vi "PilotPlant.vi"() -> ()   [LabVIEW 2019]
uses:
  Manual or Auto.ctl
  setpoints.ctl
  backwash.ctl
  coag.ctl
  model type.ctl
  data channels.ctl
  file paths.ctl
  state.ctl
  data ave state.ctl
  ini.ctl
  Sensor buffer command.ctl
  data buffer cmd.ctl
  <vilib>/addons/control/pid/pid.llb/PID (DBL).vi
  <vilib>/addons/control/pid/NI_PID_pid.lvlib
panel:
  in  "Tab Control":enum32{"Graphs", "Controls", "About"}(tab)
  in  "data points to display":u16=100 min=1 step=1
  out "coag":cluster{timestamp[], dbl[]}[](graph)
  out "Misc":cluster{timestamp[], dbl[]}[](graph)
  out "Turbidities":cluster{timestamp[], dbl[]}[](graph)
  out "Sludge valve":dbl(graph)
  out "Plant flow valve":dbl(graph)
  in  "data channel":T1
  out "recent data":dbl[](array[numeric])
  out "out of range":bool
  in  "setpoints":T2={"data update interval (s)"=100.0, "sludge flow [L/s]"=0.0, "plant flow [L/s]"=0.05, "Plant Flow PID "={"proportional gain (Kc)"=0.05, "integral time (Ti, min)"=1.0, "derivative time (Td, min)"=0.01}, "Sludge PID "={"proportional gain (Kc)"=0.07, "integral time (Ti, min)"=1.0, "derivative time (Td, min)"=0.01}, "backwash"={"Filtered quality target [NTU]"=0.3, "min filtration time [s]"=600.0, "Ripen time [s]"=600.0}, "Coagulant"={"flocculator volume (L)"=0.0, "clarifier volume (L)"=0.0, "dose updates per response delay"=100, "target clarified turbidity (NTU)"=0.3, "Coagulant mode"=enum."manual", "Coag dose [mg/L]"=0.0, "pump mL/rev"=0.0, "clarifier flow [L/s]"=0.5, "min Coag dose [mg/L]"=0.0, "max Coag dose [mg/L]"=0.0, "Steps"=3, "HRT response delay"=1, "kpf"=1.0, "DOM coag demand [mg/L]"=0.0, "min DOM coag demand [mg/L]"=0.0, "max DOM coag demand [mg/L]"=0.0}} {"Coagulant"."max DOM coag demand [mg/L]" min=0.0 max=20.0 step=0.1; "Coagulant"."min DOM coag demand [mg/L]" min=0.0 max=10.0 step=0.1; "Coagulant"."DOM coag demand [mg/L]" min=0.0 max=20.0 step=0.1; "Coagulant"."HRT response delay" min=1 max=10 step=1; "Coagulant"."Steps" min=3 step=1; "Coagulant"."clarifier flow [L/s]" min=0.0001 max=1.0 step=0.0001; "Coagulant"."target clarified turbidity (NTU)" min=0.1 max=5.0 step=0.01; "Coagulant"."dose updates per response delay" min=1 max=100 step=1; "Sludge PID"."derivative time (Td, min)" format="%.3f"; "Sludge PID"."integral time (Ti, min)" format="%.3f"; "Sludge PID"."proportional gain (Kc)" format="%.3f"; "Plant Flow PID"."derivative time (Td, min)" format="%.3f"; "Plant Flow PID"."integral time (Ti, min)" format="%.3f"; "Plant Flow PID"."proportional gain (Kc)" format="%.3f"; "plant flow [L/s]" min=0.05 max=1.0 step=0.05; "sludge flow [L/s]" min=0.0 max=0.05 step=0.001; "data update interval (s)" min=1 max=30 step=1}
  in  "Sludge valve [V]":dbl(slide)=1.5 scale=0.0..5.0
  in  "Sludge control":bool
  out "coag pump In Range?":bool
  in  "backwash [ON/OFF]":bool
  out "Last backwash":timestamp
  in  "Backwash control":T6
  out "error out":errorcluster
  out "total HRT since startup":dbl
  out "coag dose [mg/L]":dbl
  out "rpm":dbl
  out "HRT (s)":dbl
  out "Version":string
  in  "Delete buffered data":bool
  in  "channel":T1=enum."raw [NTU]"
  out "stopping":bool
  out "data labels":string[](array[string])
  in  "Shut Down":bool
  # "coag dose gets updated (dose updates per response delay). This can be a large number like 10 or 100.\nDOM coag demand updates every HRT response delay. This is the slow correction to our running estimate of the DOM\nData Buffer HRT has values stored for every coag dose update\nThe coagulant update code is at most called every data update interval, so make sure that the data interval is faster than the dose updates per response delay.\ndata update interval has a maximum value of 30 seconds to ensure that  it is much smaller than the HRT."
  # "ramp controls"
  # "min"
  # "max"
  # "min"
  # "max"
  # "The coaglog saves the coagulant and turbidity values for that particular time. There is no offset to correct for HRT.\ncoagulant demand at time t was calculated based on data from HRT response delay ago.\n\nhttps://aguaclara.github.io/Textbook/Operation/Coagulant_Automation.html\n\nAguaClara Textbook v1.4.27"
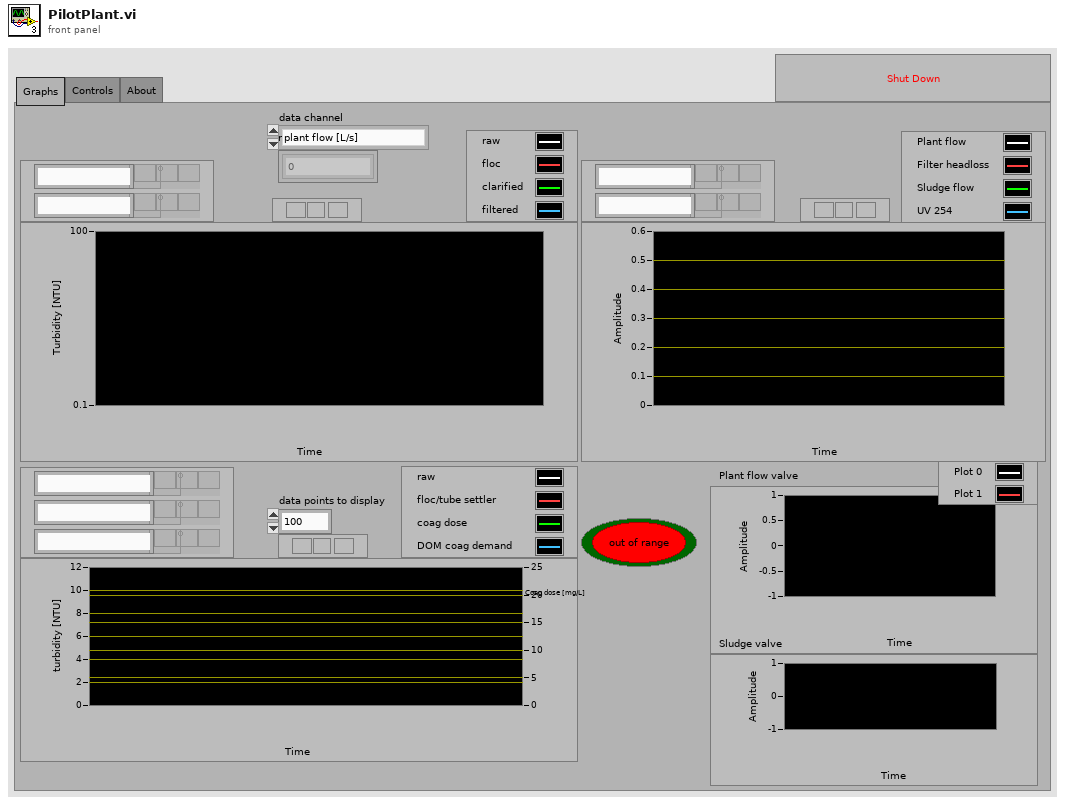
[diagram p1: front panel]
types:
  T1 = typedef "data channels.ctl" = enum16{"plant flow [L/s]", "Head Loss [m]", "sludge flow [L/s]", "UV 254", "raw [NTU]", "floc sed [NTU]", "clarified [NTU]", "filtered [NTU]"}
  T2 = typedef "setpoints.ctl" = cluster{"data update interval (s)":sgl, "sludge flow [L/s]":dbl, "plant flow [L/s]":dbl, "Plant Flow PID ":cluster{"proportional gain (Kc)":dbl, "integral time (Ti, min)":dbl, "derivative time (Td, min)":dbl}, "Sludge PID ":cluster{"proportional gain (Kc)":dbl, "integral time (Ti, min)":dbl, "derivative time (Td, min)":dbl}, "backwash":T3, "Coagulant":T4}
  T3 = typedef "backwash.ctl" = cluster{"Filtered quality target [NTU]":dbl, "min filtration time [s]":dbl, "Ripen time [s]":dbl}
  T4 = typedef "coag.ctl" = cluster{"flocculator volume (L)":dbl, "clarifier volume (L)":dbl, "dose updates per response delay":u16, "target clarified turbidity (NTU)":dbl, "Coagulant mode":T5, "Coag dose [mg/L]":dbl, "pump mL/rev":dbl, "clarifier flow [L/s]":dbl, "min Coag dose [mg/L]":dbl, "max Coag dose [mg/L]":dbl, "Steps":u16, "HRT response delay":u32, "kpf":dbl, "DOM coag demand [mg/L]":dbl, "min DOM coag demand [mg/L]":dbl, "max DOM coag demand [mg/L]":dbl}
  T5 = typedef "model type.ctl" = enum16{"manual", "ramp", "simple corrector"}
  T6 = typedef "Manual or Auto.ctl" = enum16{"Manual", "Automatic"}
  T7 = typedef "state.ctl" = enum16{"Initialize", "Process data", "Close"}
  T8 = typedef "file paths.ctl" = enum16{"read paths", "close"}
  T9 = typedef "ini.ctl" = enum16{"write", "read"}
  T10 = typedef "data ave state.ctl" = enum16{"Initialize", "Process data"}
  T11 = typedef "data buffer cmd.ctl" = enum16{"set buffer size", "write", "refill buffer", "read recent", "read all", "clear"}
  T12 = typedef "Sensor buffer command.ctl" = enum16{"set buffer size", "write", "refill buffer", "read recent", "read all", "read at delta HRT", "clear"}
  T13 = cluster{"proportional gain (Kc)":dbl, "integral time (Ti, min)":dbl, "derivative time (Td, min)":dbl}
  T14 = typedef "data cluster.ctl" = cluster{"floc sed turbidity (NTU)":dbl, "Raw turbidity (NTU)":dbl, "flow rate (L/s)":dbl, "time":timestamp, "Cumulative HRT":dbl, "Coag dose (mg/L)":dbl, "DOM coag demand (mg/L)":dbl, "DOM in range":bool, "update DOM":bool}
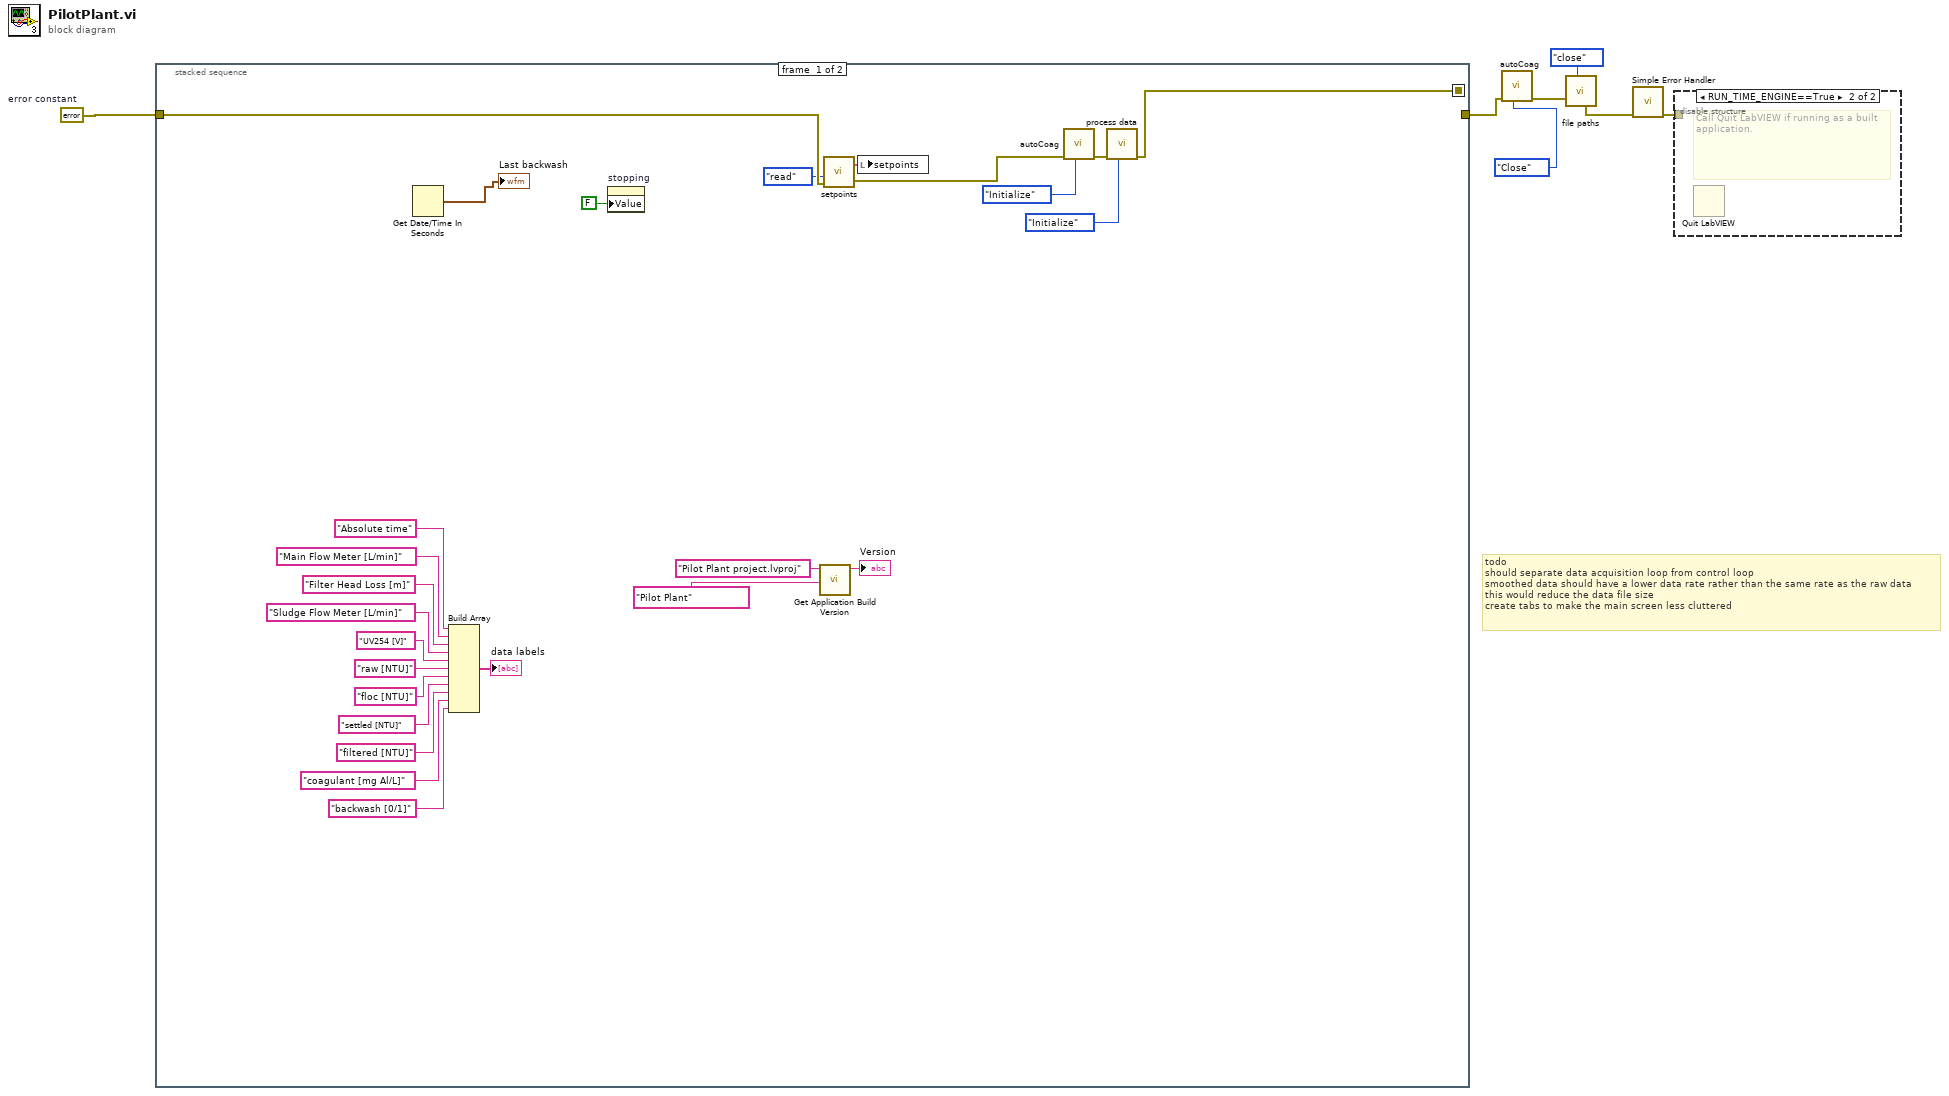
[diagram p0: block diagram]
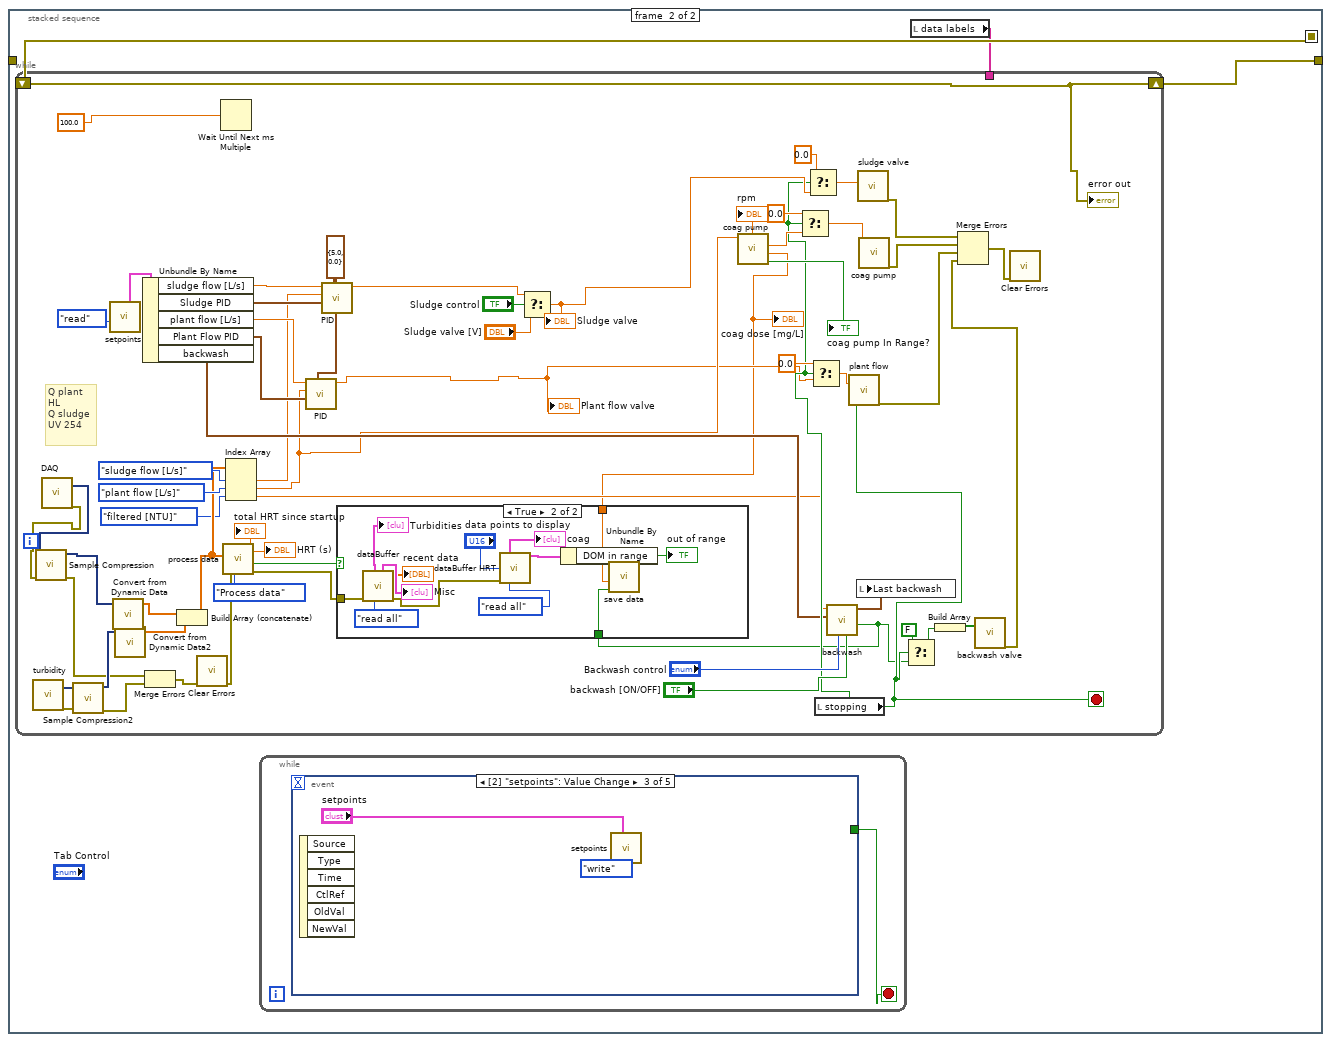
[diagram p2: hidden frame]
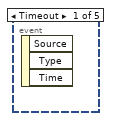
[diagram p3: hidden frame]
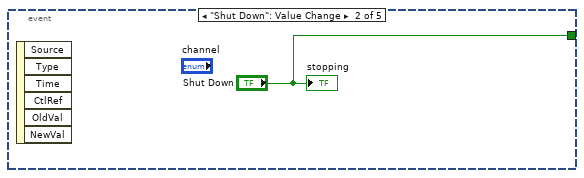
[diagram p4: hidden frame]
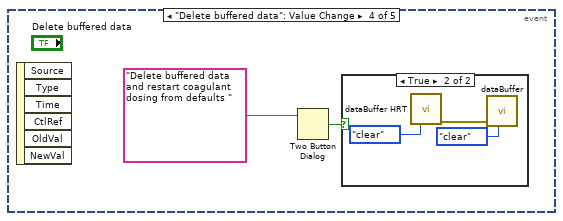
[diagram p5: hidden frame]
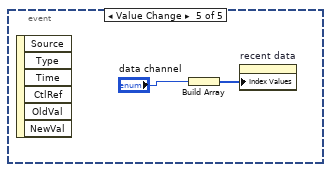
[diagram p7: hidden frame]
diagram:
  w7 = errorcluster {"status"=FALSE, "code"=0, "source"=""}  # error constant
  # "todo\nshould separate data acquisition loop from control loop\nsmoothed data should have a lower data rate rather than the same rate as the raw data\nthis would reduce the data file size\ncreate tabs to make the main screen less cluttered"
  n1 = stacked-sequence {
    seq-local: [w15 _] -> [_ w35]
    tunnel: w7 -> [w13 _]
    tunnel: [_ w33] -> w2
    frame #0 {
      n2 = Get Date/Time In Seconds() -> (seconds since 1Jan1904=→"Last backwash":timestamp)
      n3 = Build Array("Absolute time", "Main Flow Meter [L/min]", "Filter Head Loss [m]", "Sludge Flow Meter [L/min]", "UV254 [V]" ("element"), "raw [NTU]", "floc [NTU]", "settled [NTU]", "filtered [NTU]" ("element"), "coagulant [mg Al/L]" ("element"), "backwash [0/1]" ("element")) -> (→"data labels":string[])
      n4 = property on="stopping" class="Bool (strict)"("Value"=FALSE ("stopping")) -> ()  [unwired: 2 in, 2 out]
      n5 = call "Get Application Build Version.vi"("Build Specification Name"="Pilot Plant", "Project Filename"="Pilot Plant project.lvproj") -> ("Version String"=→"Version":string)  [unwired: 7 in, 2 out]
      n6 = call "setpoints.vi"("error in (no error)"=w13, "ini"=ini."read") -> ("error out"=w12:errorcluster, "Setpoints out"=w14:T2)  [unwired: 8 in]
      n7 = local write "setpoints"(w14) -> ()
      n8 = call "autoCoag.vi"("state"=state."Initialize" ("Enum"), "error in (no error)"=w12) -> ("error out"=w17:errorcluster)  [unwired: 7 in, 2 out]
      n9 = call "process data.vi"("state"=data_ave_state."Initialize", "error in (no error)"=w17) -> ("error out"=w15:errorcluster)  [unwired: 5 in, 4 out]
    }
    frame #1 {
      n10 = while {
        stop <- w36 stop-if-true
        n11 = event shown="[2] \"setpoints\": Value Change" {
          selector: _ -> [_ _ _ _ _]
          dyn-events: _ -> [_ _ _ _ _]
          timeout: _ -> [_ _ _ _ _]
          tunnel: [_ "Shut Down" _ _ _] -> w36
          event Timeout {
            n12 = event-data() -> ()  [unwired: 1 in, 3 out]
          }
          event "Shut Down": Value Change {
            n13 = event-data() -> ()  [unwired: 1 in, 6 out]
            "stopping" <- "Shut Down"
          }
          event Value Change {
            n14 = event-data() -> ()  [unwired: 1 in, 6 out]
            n15 = call "setpoints.vi"("setpoints"="setpoints", "ini"=ini."write") -> ()  [unwired: 8 in, 2 out]
          }
          event "Delete buffered data": Value Change {
            n16 = event-data() -> ()  [unwired: 1 in, 6 out]
            n17 = Two Button Dialog(message="Delete buffered data and restart coagulant dosing from defaults ") -> (T button?=w40:bool)  [unwired: 2 in]
            n18 = case shown="True" w40 {
              frame False {
              }
              frame True {
                n19 = call "dataBuffer HRT.vi"("command"=Sensor_buffer_command."clear") -> ("error out"=w42:errorcluster)  [unwired: 9 in, 5 out]
                n20 = call "dataBuffer.vi"("command"=data_buffer_cmd."clear", "error in (no error)"=w42) -> ()  [unwired: 4 in, 6 out]
              }
            }
          }
          event Value Change {
            n21 = event-data() -> ()  [unwired: 1 in, 6 out]
            n22 = Build Array("data channel") -> (w45:T1[])
            n23 = property on="recent data" class="Arr (strict)"("Index Values"=w45) -> ()  [unwired: 2 in, 2 out]
          }
        }
      }
      n24 = local read "data labels"() -> (w34:string[])
      n25 = while {
        shift-right: [w73] -> w33
        shift-left: w35 -> [w73]
        tunnel: w34 -> [_]
        stop <- w90 stop-if-true
        w103 = cluster{"output high":dbl, "output low":dbl} {"output high"=5.0, "output low"=0.0} ("output range")
        # "Q plant\nHL\nQ sludge\nUV 254"
        n26 = call "turbidity"() -> ("data"=w76:dynamicdata, "error out"=w58:errorcluster)  [unwired: 17 in, 1 out]
        n27 = call "DAQ"() -> ("data"=w77:dynamicdata, "error out"=w59:errorcluster)  [unwired: 17 in, 1 out]
        n28 = call "Sample Compression"("error in (no error)"=w59, "Signals"=w77) -> ("error out"=w57:errorcluster, "Mean"=w72:dynamicdata)  [unwired: 7 in, 1 out]
        n29 = call "Sample Compression2"("error in (no error)"=w58, "Signals"=w76) -> ("error out"=w56:errorcluster, "Mean"=w67:dynamicdata)  [unwired: 7 in, 1 out]
        n30 = call "setpoints.vi"("ini"=ini."read") -> ("Setpoints out"=w74:T2)  [unwired: 9 in, 1 out]
        n31 = call "Convert from Dynamic Data"("Dynamic Data Type"=w72) -> ("Array"=w88:dbl[])  [unwired: 3 in]
        n32 = call "Convert from Dynamic Data2"("Dynamic Data Type"=w67) -> ("Array"=w87:dbl[])  [unwired: 3 in]
        n33 = Unbundle By Name(w74) -> ("sludge flow [L/s]"=w83:dbl, "Sludge PID"=w82:T13, "plant flow [L/s]"=w81:dbl, "Plant Flow PID"=w80:T13, "backwash"=w79:T3)
        n34 = Merge Errors(w57, w56) -> (w55:errorcluster)
        n35 = Build Array (concatenate)(w88, w87) -> (w66:dbl[])
        n36 = call <vilib>:"Clear Errors.vi"("error in (no error)"=w55) -> ("error out"=w54:errorcluster)  [unwired: 5 in, 1 out]
        n37 = Wait Until Next ms Multiple(millisecond multiple=100.0 ("y")) -> ()  [unwired: 1 out]
        n38 = call "process data.vi"("state"=data_ave_state."Process data", "error in (no error)"=w54, "data input"=w66) -> ("error out"=w53:errorcluster, "new interval"=w84:bool, "total HRT"=→"total HRT since startup":dbl, "HRT (s)"=→"HRT (s)":dbl)  [unwired: 4 in, 1 out]
        n39 = Index Array(array=w66, index #1=data_channels."sludge flow [L/s]" ("channel"), index #2=data_channels."plant flow [L/s]" ("channel"), index #3=data_channels."filtered [NTU]" ("channel")) -> (element #1=w69:dbl, element #2=w68:dbl, element #3=w64:dbl)
        n40 = call-poly <vilib>:"PID.vi"("output range"=w103, "PID gains"=w80, "process variable"=w68, "setpoint"=w81) -> ("output"=w62:dbl)  [unwired: 6 in, 1 out]
        "Plant flow valve" <- w62
        n41 = call-poly <vilib>:"PID.vi"("output range"=w103, "PID gains"=w82, "process variable"=w69, "setpoint"=w83) -> ("output"=w104:dbl)  [unwired: 6 in, 1 out]
        n42 = Select(t=w104, s="Sludge control", f="Sludge valve [V]") -> (s? t:f=w94:dbl)
        "Sludge valve" <- w94
        n43 = call "coag pump.vi"("plant flow [L/s]"=w68) -> ("In Range?"=→"coag pump In Range?":bool, "coag dose [mg/L]"=w47:dbl, "pump [V]"=w99:dbl, "rpm"=→"rpm":dbl)  [unwired: 6 in, 1 out]
        "coag dose [mg/L]" <- w47
        n44 = local read "stopping"() -> (w90:bool)
        n45 = Select(t=0.0, s=w90, f=w99) -> (s? t:f=w98:dbl)
        n46 = Select(t=0.0, s=w90, f=w94) -> (s? t:f=w93:dbl)
        n47 = Select(t=0.0, s=w90, f=w62) -> (s? t:f=w97:dbl)
        n48 = call "backwash.vi"("Manual override"="backwash [ON/OFF]", "Backwash control"="Backwash control", "backwash"=w79, "Filtered Turbidity"=w64) -> ("backwashing?"=w63:bool, "last backwash"=w105:timestamp)  [unwired: 5 in, 1 out]
        n49 = case shown="True" w84 {
          tunnel: w47 -> [_ w120]
          tunnel: w63 -> [_ w119]
          tunnel: w53 -> [_ w113]
          frame False {
          }
          frame True {
            n50 = call "dataBuffer.vi"("command"=data_buffer_cmd."read all", "error in (no error)"=w113) -> ("error out"=w112:errorcluster, "recent data"=→"recent data":dbl[], "misc graph"=→"Misc":cluster{timestamp[], dbl[]}[], "turbidity"=→"Turbidities":cluster{timestamp[], dbl[]}[])  [unwired: 4 in, 2 out]
            n51 = call "dataBuffer HRT.vi"("data to display"="data points to display", "error in (no error)"=w112, "command"=Sensor_buffer_command."read all") -> ("coag graph"=→"coag":cluster{timestamp[], dbl[]}[], "recent data"=w110:T14)  [unwired: 7 in, 4 out]
            n52 = Unbundle By Name(w110) -> ("DOM in range"=→"out of range":bool)
            n53 = call "save data.vi"("backwashing?"=w119, "coagulant dose"=w120) -> ()  [unwired: 10 in]
          }
        }
        n54 = call "plant flow"("data"=w97, "stop (T)"=w90) -> ("error out"=w50:errorcluster)  [unwired: 16 in, 1 out]
        n55 = local write "Last backwash"(w105) -> ()
        n56 = call "sludge valve"("data"=w93) -> ("error out"=w52:errorcluster)  [unwired: 17 in, 1 out]
        n57 = call "coag pump"("data"=w98) -> ("error out"=w51:errorcluster)  [unwired: 17 in, 1 out]
        n58 = Select(t=FALSE, s=w90, f=w63) -> (s? t:f=w91:bool)
        n59 = Build Array(w91) -> (w108:bool[])
        n60 = call "backwash valve"("data"=w108) -> ("error out"=w49:errorcluster)  [unwired: 17 in, 1 out]
        n61 = Merge Errors(w52, w51, w50, w49) -> (w48:errorcluster)
        n62 = call <vilib>:"Clear Errors.vi"("error in (no error)"=w48) -> ()  [unwired: 5 in, 2 out]
        "error out" <- w73
      }
    }
  }
  n63 = call "autoCoag.vi"("state"=state."Close" ("Enum"), "error in (no error)"=w2) -> ("error out"=w1:errorcluster)  [unwired: 7 in, 2 out]
  n64 = call "file paths.vi"("error in (no error)"=w1, "file path control"=file_paths."close") -> ("error out"=w4:errorcluster)  [unwired: 6 in, 3 out]
  n65 = call <vilib>:"Simple Error Handler.vi"("error in (no error)"=w4) -> ("error out"=w6:errorcluster)  [unwired: 4 in, 4 out]
  n66 = disable-structure shown="RUN_TIME_ENGINE==True" {
    disable-tunnel: w6 -> [_ _]
    frame condition #0 (active) {
    }
    frame condition #1 {
      # "Call Quit LabVIEW if running as a built application."
      n67 = Quit LabVIEW() -> ()  [unwired: 1 in]
    }
  }
